vi "Change Column Units.vi"(6 "Change units":string, 8 "error in (no error)":errorcluster, 9 "selected column path":string, 10 "selected table path":string, 11 "Data.PG in":refnum<class "LV-Data.PGSQL.lvclass">) -> (0 "error out":errorcluster, 3 "Data.PG out":refnum<class "LV-Data.PGSQL.lvclass">)   [LabVIEW 2019, in "LV-Data.PGSQL.lvclass"]
uses:
  LV-Data.PGSQL.lvclass
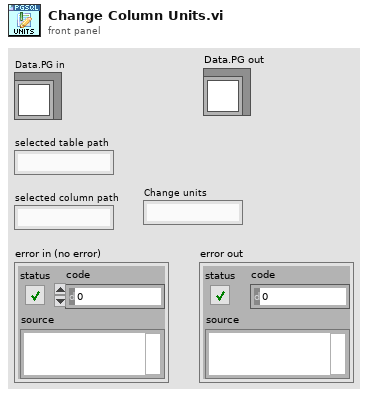
[diagram p1: front panel]
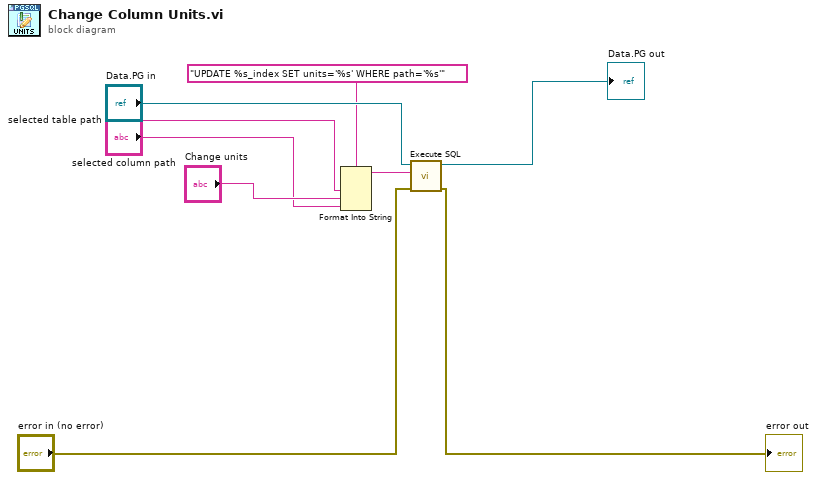
[diagram p0: block diagram]
diagram:
  n1 = Format Into String(format string="UPDATE %s_index SET units='%s' WHERE path='%s'", "selected table path", "Change units", "selected column path") -> (resulting string=w2:string)  [unwired: 2 in, 1 out]
  n2 = call "Execute SQL.vi"("error in"="error in (no error)", "SQL"=w2, "LV-Data.PGSQL"="Data.PG in") -> ("error out"=→"error out":errorcluster, "LV-Data.PGSQL out"=→"Data.PG out":refnum<class "LV-Data.PGSQL.lvclass">)  [unwired: 5 in, 2 out]
